vi "习题7.4.vi"() -> ()   [LabVIEW 2017]
panel:
  in  "停止":bool
  in  "可见":bool
  out "波形图":dbl[](graph)
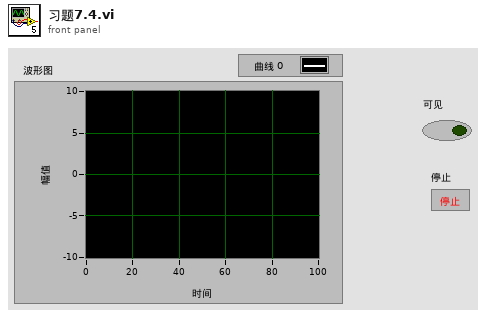
[diagram p1: front panel]
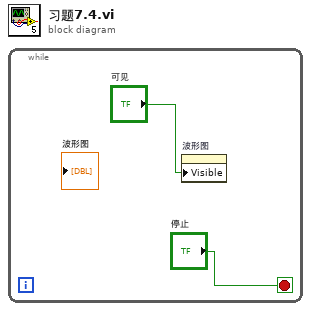
[diagram p0: block diagram]
diagram:
  n1 = while {
    stop <- "停止" stop-if-true
    n2 = property on="波形图" class="WFGraph (严格)"("Visible"="可见") -> ()  [unwired: 2 in, 2 out]
  }
